vi "Untitled 1.vi"() -> ()   [LabVIEW 2024]
panel:
  in  "Login 8":bool
  in  "Side Left":T1
  in  "Login 6":bool
  in  "Login 7":bool
  in  "Tab Control":T2(tab)
  in  "Password":string
  in  "Username":string(combo)
  in  "Login":bool
  in  "Login 5":bool
  in  "Login 4":bool
  in  "Login 3":bool
  in  "Login 2":bool
  in  "Tab Control 2":enum32{"Batch select", "Roller", "Dashboard"}(tab)
  in  "Batch CB":string(combo)
  out "String 2":string
  out "Waveform Graph":dbl[](graph)
  in  "Setting":bool
  in  "Setting 2":bool
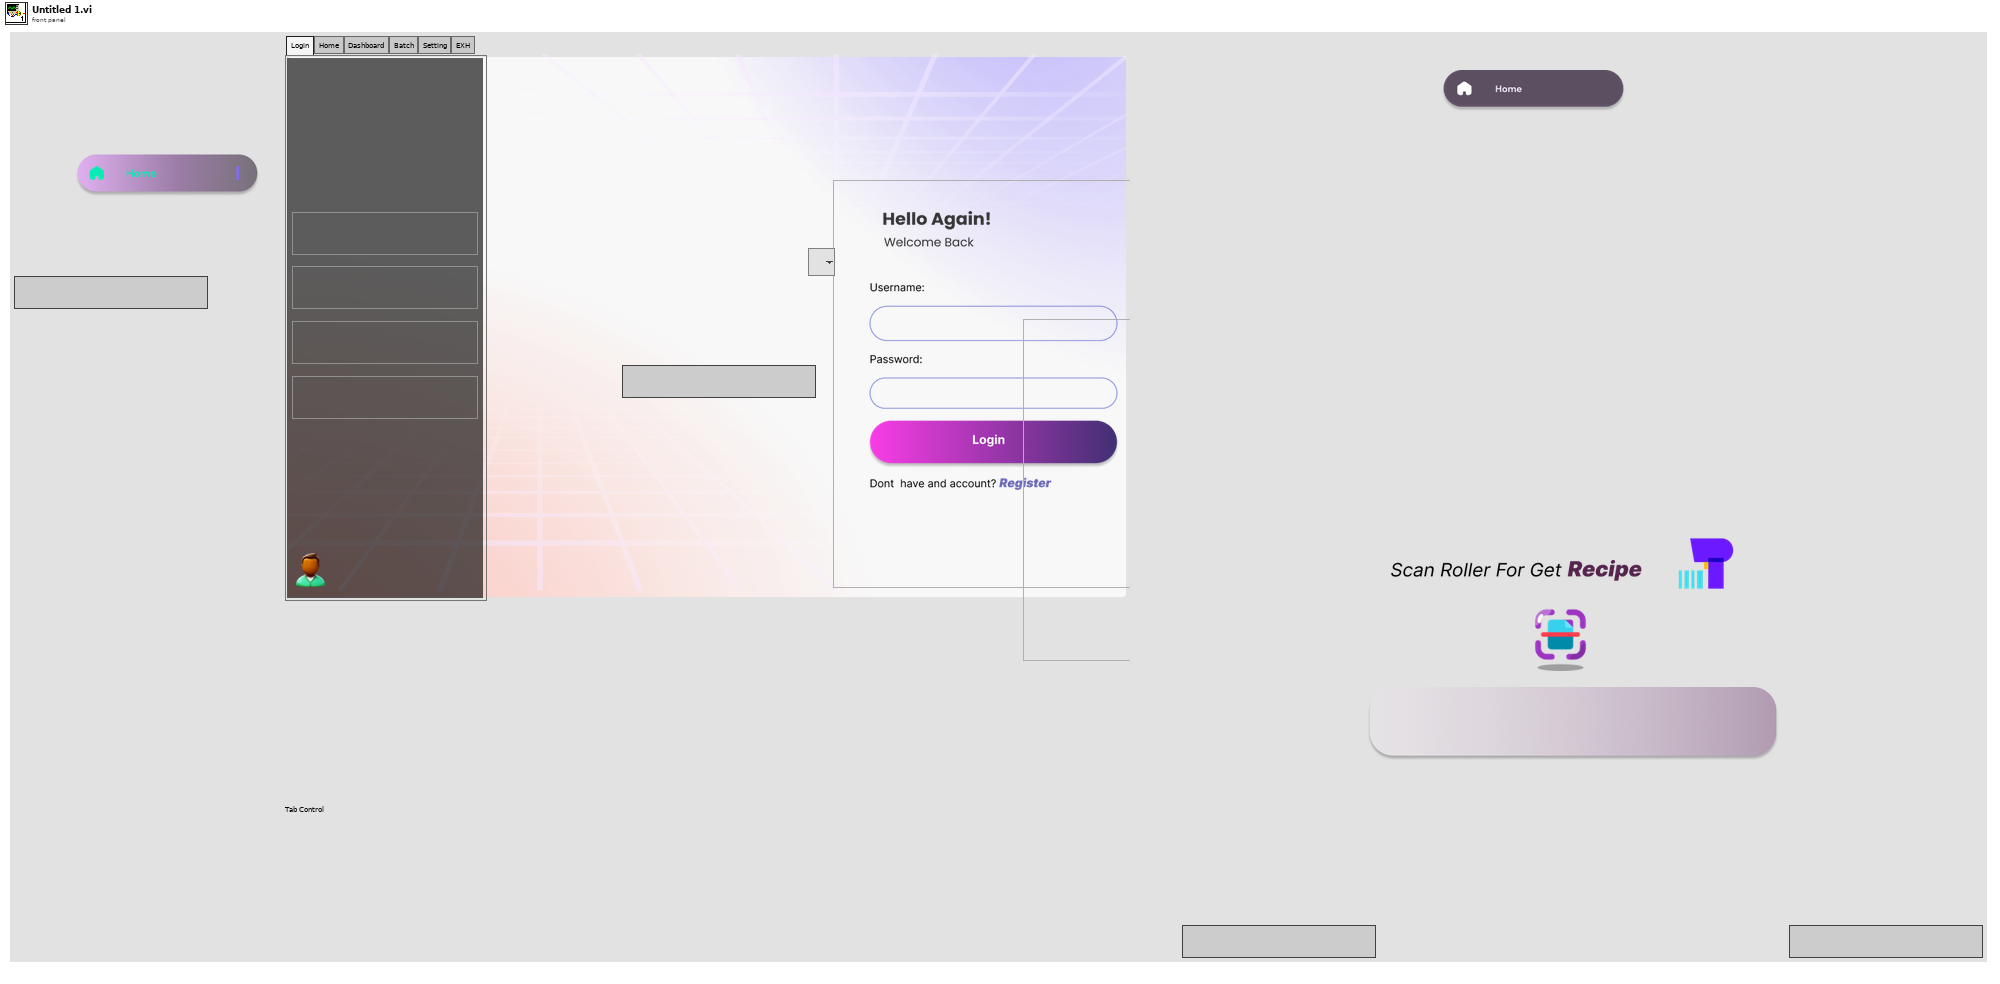
[diagram p1: front panel]
types:
  T1 = cluster{"Home":bool, "Dashboard":bool, "Setting":bool, "EXH":bool}
  T2 = enum32{"Login", "Home", "Dashboard", "Batch", "Setting", "EXH"}
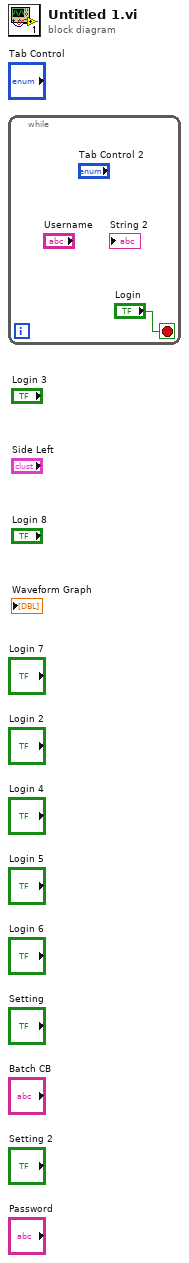
[diagram p0: block diagram]
diagram:
  n1 = while {
    stop <- "Login" stop-if-true
  }
